vi "stopGrab.vi"(8 "error in (no error)":errorcluster, 11 "camera in":refnum<class "camera.lvclass">) -> (0 "error out":errorcluster, 3 "camera out":refnum<class "camera.lvclass">)   [LabVIEW 2017, in "camera.lvclass"]
uses:
  camera.lvclass
  <vilib>/vision/driver/NI_Vision_Acquisition_Software.lvlib
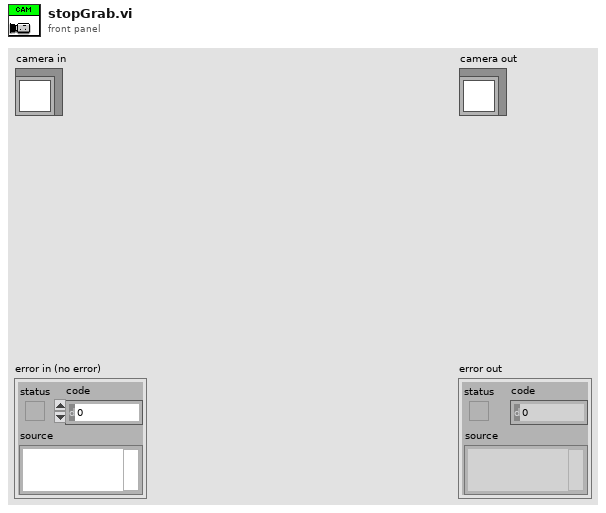
[diagram p1: front panel]
types:
  T1 = typedef "IMAQdx.ctl" = refnum<k21>
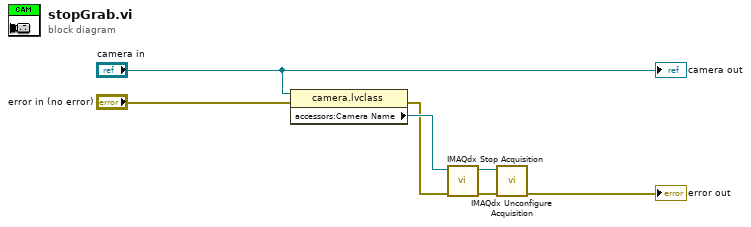
[diagram p0: block diagram]
diagram:
  n1 = property class="camera.lvclass"(reference="camera in", error in="error in (no error)") -> (error out=w3:errorcluster, "accessors:Camera Name"=w4:refnum<k21>)  [unwired: 1 out]
  n2 = call <vilib>:"IMAQdx Stop Acquisition.vi"("error in"=w3, "Session In"=w4) -> ("error out"=w5:errorcluster, "Session Out"=w6:T1)  [unwired: 8 out]
  n3 = call <vilib>:"IMAQdx Unconfigure Acquisition.vi"("error in"=w5, "Session In"=w6) -> ("error out"=→"error out":errorcluster)  [unwired: 9 out]
  "camera out" <- "camera in"
